vi "HEWH Get Excel Data.vi"   [LabVIEW 2019]
uses:
  <vilib>/addons/_office/NI_ReportGenerationToolkit.lvlib
  <vilib>/addons/_office/excel.llb/Excel Easy Table (str).vi
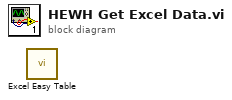
[diagram p0: block diagram]
diagram:
  n1 = call-poly <vilib>:"Excel Easy Table.vi"() -> ()  [unwired: 11 in, 5 out]
